vi "delta_time.vi"(6 "Time in":dbl, 9 "error in (no error)":errorcluster) -> (1 "error out":errorcluster, 2 "Delta Time":dbl, 4 "Time out":dbl)   [LabVIEW 2024]
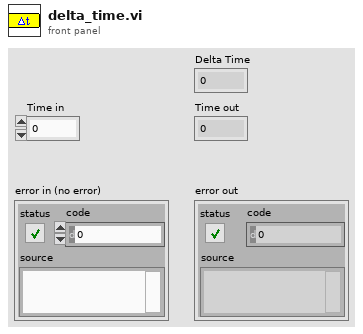
[diagram p1: front panel]
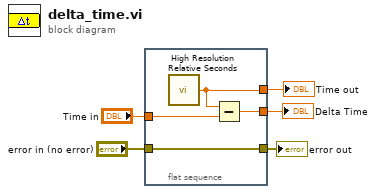
[diagram p0: block diagram]
diagram:
  n1 = flat-sequence {
    tunnel: [w9] -> w5
    tunnel: "error in (no error)" -> [w9]
    tunnel: "Time in" -> [w8]
    tunnel: [w7] -> w2
    tunnel: [w6] -> w1
    frame #0 {
      n2 = call <vilib>:"High Resolution Relative Seconds.vi"() -> ("relative seconds"=w7:dbl)
      n3 = Subtract(x=w7, y=w8) -> (x-y=w6:dbl)
    }
  }
  "error out" <- w5
  "Time out" <- w2
  "Delta Time" <- w1
